vi "save_spectroscopy_hdf.vi"(3 "System Information cluster":T1, 5 "Subject metadata cluster":T2, 7 "Device Name":tag="DAQ2", 8 "Spectroscopy cluster in":T4, 9 "TxRxParams":T3={"sample rate"=1000000.0, "Transmit frequency"=25000.0, "Transmit amplitude"=1.577, "sample rate digital out"=40000.0, "TX cycles"=600, "sample rate DAQ1"=1000000.0, "Receive frequency"=75000.0, "Receive range"=1.0, "TX harmonics"=[50000.0, 75000.0, 100000.0, 125000.0, 150000.0, 175000.0, 200000.0, 225000.0]} {"TX harmonics" format="%#_6p"; "Receive frequency" format="%#_6p"; "sample rate DAQ1" format="%#_6p"; "sample rate digital out" format="%#_6p"; "Transmit frequency" format="%#_6p"; "sample rate" format="%#_6p"}, 11 "file path":path) -> ()   [LabVIEW 2021]
uses:
  <vilib>/UPVI/lvhdf5/file.llb/LVH5F Operation.ctl
  <vilib>/Utility/miscctls.llb/LVRectTypeDef.ctl
  <vilib>/UPVI/lvhdf5/group.llb/H5G_obj_t.ctl
  <vilib>/UPVI/lvhdf5/dataset.llb/LVH5D Operation.ctl
  <vilib>/UPVI/lvhdf5/attribute.llb/LVH5A Operation.ctl
  <vilib>/UPVI/lvhdf5/identifier.llb/Not an HDF5 Refnum Constant.vi
  <vilib>/UPVI/lvhdf5/attribute.llb/Write Multiple Attributes.vi
  <vilib>/UPVI/lvhdf5/utility.llb/Select HDF5 Dialog.vi
  <vilib>/UPVI/lvhdf5/utility.llb/Select HDF5 Dialog (Object Only).vi
  <vilib>/UPVI/lvhdf5/dataset.llb/Simple H5Dwrite (Variant).vi
  <vilib>/UPVI/lvhdf5/common.llb/To HDF5 Ref.vi
  <vilib>/UPVI/lvhdf5/dataset.llb/H5Dclose.vi
  <vilib>/UPVI/lvhdf5/attribute.llb/Simple H5Awrite (Variant).vi
  <vilib>/UPVI/lvhdf5/attribute.llb/LVH5 Write Attributes.xnode
  <vilib>/UPVI/lvhdf5/library.llb/HDF5 Ref.ctl
  <vilib>/UPVI/lvhdf5/dataset.llb/Simple H5Dwrite.xnode
  <vilib>/UPVI/lvhdf5/dataset.llb/Write Dataset with Attributes.xnode
  <vilib>/UPVI/lvhdf5/attribute.llb/Simple H5Awrite.xnode
  <vilib>/UPVI/lvhdf5/attribute.llb/Cluster to Attribute Array.xnode
  <vilib>/Utility/error.llb/Error Cluster From Error Code.vi
  <vilib>/UPVI/lvhdf5/dataset.llb/OpenCreateReplace Dataset by Element Type.vi
  <vilib>/UPVI/lvhdf5/dataspace.llb/H5Sselect_hyperslab.vi
  <vilib>/UPVI/lvhdf5/dataset.llb/H5Dwrite (Variant).vi
  <vilib>/UPVI/lvhdf5/dataset.llb/H5Dget_space.vi
  <vilib>/UPVI/lvhdf5/attribute.llb/private/LVH5AwriteWDTAttrs.vi
  <vilib>/UPVI/lvhdf5/dataspace.llb/H5Sclose.vi
  <vilib>/UPVI/lvhdf5/utility.llb/Select HDF5 Dialog (File and Object).vi
  <resource>/objmgr/daqmx.rc
  <vilib>/UPVI/lvhdf5/library.llb/HDF5 Ref.lvclass
  <vilib>/Utility/Data Type/Get Type Information.vi
  <vilib>/Utility/Data Type/NI_Data Type.lvlib
  <vilib>/Utility/Data Type/Get Cluster Information.vi
panel:
  out "proj mag f2-f9":dbl[][](array[numeric])
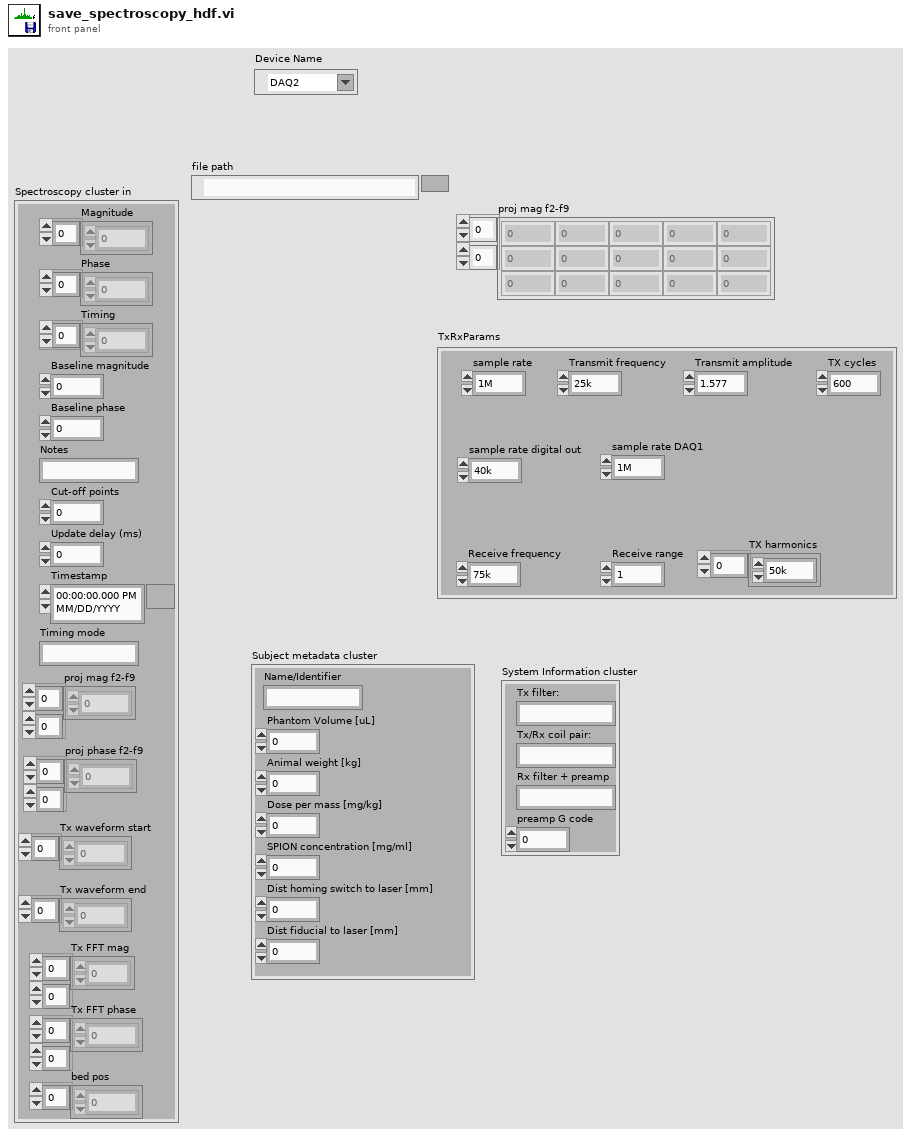
[diagram p1: front panel]
types:
  T1 = cluster{"Tx filter:":string, "Tx/Rx coil pair:":string, "Rx filter + preamp":string, "preamp G code":dbl}
  T2 = cluster{"Name/Identifier":string, "Phantom Volume [uL]":dbl, "Animal weight [kg]":dbl, "Dose per mass [mg/kg]":dbl, "SPION concentration [mg/ml]":dbl, "Dist homing switch to laser [mm]":dbl, "Dist fiducial to laser [mm]":dbl}
  T3 = cluster{"sample rate":dbl, "Transmit frequency":dbl, "Transmit amplitude":dbl, "sample rate digital out":dbl, "TX cycles":i32, "sample rate DAQ1":dbl, "Receive frequency":dbl, "Receive range":dbl, "TX harmonics":dbl[]}
  T4 = cluster{"Magnitude":dbl[], "Phase":dbl[], "Timing":dbl[], "Baseline magnitude":dbl, "Baseline phase":dbl, "Notes":string, "Cut-off points":i32, "Update delay (ms)":dbl, "Timestamp":timestamp, "Timing mode":string, "proj mag f2-f9":dbl[][], "proj phase f2-f9":dbl[][], "Tx waveform start":dbl[], "Tx waveform end":dbl[], "Tx FFT mag":dbl[][], "Tx FFT phase":dbl[][], "bed pos":dbl[]}
  T5 = typedef "LVH5F Operation.ctl" = enum16{"open", "open or create", "create or replace", "create or replace (with confirmation)", "create", "open (read only)"}
  T6 = typedef "HDF5 Ref.ctl" = refnum<class "HDF5 Ref.lvclass">
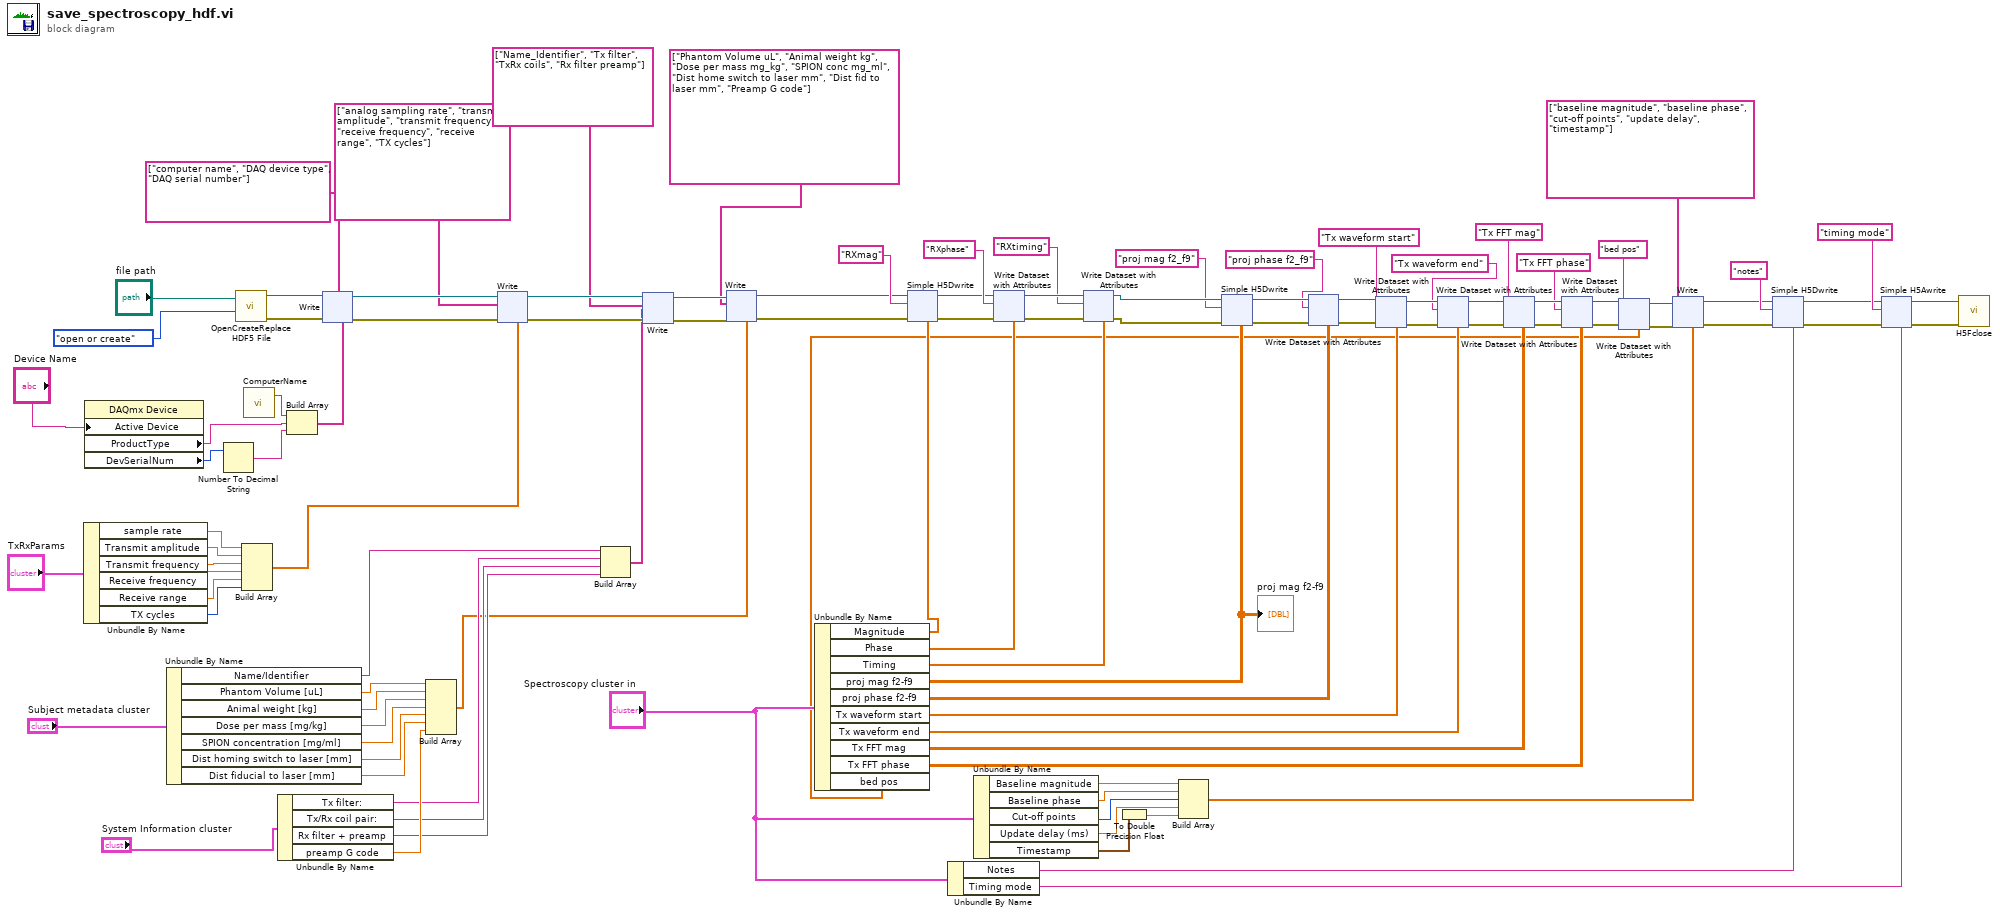
[diagram p0: block diagram]
diagram:
  n1 = Unbundle By Name("TxRxParams") -> ("sample rate"=w24:dbl, "Transmit amplitude"=w25:dbl, "Transmit frequency"=w26:dbl, "Receive frequency"=w27:dbl, "Receive range"=w28:dbl, "TX cycles"=w29:i32)
  n2 = property class="DAQmx Device"("Active Device"="Device Name") -> ("ProductType"=w95:string, "DevSerialNum"=w97:u32)  [unwired: 2 in, 2 out]
  n3 = Unbundle By Name("Subject metadata cluster") -> ("Name/Identifier"=w11:string, "Phantom Volume [uL]"=w17:dbl, "Animal weight [kg]"=w16:dbl, "Dose per mass [mg/kg]"=w15:dbl, "SPION concentration [mg/ml]"=w14:dbl, "Dist homing switch to laser [mm]"=w13:dbl, "Dist fiducial to laser [mm]"=w12:dbl)
  n4 = Number To Decimal String(number=w97) -> (decimal integer string=w96:string)  [unwired: 1 in]
  n5 = call <vilib>:"OpenCreateReplace HDF5 File.vi"("function (open or create)"=LVH5F_Operation."open or create", "path"="file path") -> ("error out"=w86:errorcluster, "HDF5 Ref out"=w87:T6)  [unwired: 6 in]
  n6 = Build Array(w24, w25, w26, w27, w28, w29) -> (w91:dbl[])
  n7 = call "ComputerName.vi"() -> ("String/Binary data"=w94:string)  [unwired: 4 in, 1 out]
  n8 = Unbundle By Name("System Information cluster") -> ("Tx filter:"=w9:string, "Tx/Rx coil pair:"=w8:string, "Rx filter + preamp"=w7:string, "preamp G code"=w10:dbl)
  n9 = Build Array(w94, w95, w96) -> (w93:string[])
  n10 = xnode "Write"("HDF5 Ref"=w87, "error in (no error)"=w86, "Name(s)"=string[] ["computer name", "DAQ device type", "DAQ serial number"], "Value(s)"=w93) -> ("HDF5 Ref out"=w85:T6, "error out"=w84:errorcluster)  [unwired: 1 in]
  n11 = Build Array(w17, w16, w15, w14, w13, w12, w10) -> (w3:dbl[])
  n12 = xnode "Write"("HDF5 Ref"=w85, "error in (no error)"=w84, "Name(s)"=string[] ["analog sampling rate", "transmit amplitude", "transmit frequency", "receive frequency", "receive range", "TX cycles"], "Value(s)"=w91) -> ("HDF5 Ref out"=w23:T6, "error out"=w21:errorcluster)  [unwired: 1 in]
  n13 = Build Array(w11, w9, w8, w7) -> (w4:string[])
  n14 = xnode "Write"("HDF5 Ref"=w23, "error in (no error)"=w21, "Name(s)"=string[] ["Name_Identifier", "Tx filter", "TxRx coils", "Rx filter preamp"], "Value(s)"=w4) -> ("HDF5 Ref out"=w22:T6, "error out"=w20:errorcluster)  [unwired: 1 in]
  n15 = xnode "Write"("HDF5 Ref"=w22, "error in (no error)"=w20, "Name(s)"=string[] ["Phantom Volume uL", "Animal weight kg", "Dose per mass mg_kg", "SPION conc mg_ml", "Dist home switch to laser mm", "Dist fid to laser mm", "Preamp G code"], "Value(s)"=w3) -> ("HDF5 Ref out"=w18:T6, "error out"=w19:errorcluster)  [unwired: 1 in]
  n16 = Unbundle By Name("Spectroscopy cluster in") -> ("Magnitude"=w82:dbl[], "Phase"=w81:dbl[], "Timing"=w78:dbl[], "proj mag f2-f9"=w56:dbl[][], "proj phase f2-f9"=w53:dbl[][], "Tx waveform start"=w46:dbl[], "Tx waveform end"=w45:dbl[], "Tx FFT mag"=w38:dbl[][], "Tx FFT phase"=w37:dbl[][], "bed pos"=w31:dbl[])
  "proj mag f2-f9" <- w56
  n17 = xnode "Simple H5Dwrite"("Dataset Path"="RXmag", "error in (no error)"=w19, "HDF5 Path or Ref"=w18, "Data"=w82) -> ("HDF5 Ref out"=w99:T6, "error out"=w100:errorcluster)  [unwired: 4 in, 1 out]
  n18 = Unbundle By Name("Spectroscopy cluster in") -> ("Notes"=w71:string, "Timing mode"=w65:string)
  n19 = Unbundle By Name("Spectroscopy cluster in") -> ("Baseline magnitude"=w76:dbl, "Baseline phase"=w75:dbl, "Cut-off points"=w74:i32, "Update delay (ms)"=w73:dbl, "Timestamp"=w64:timestamp)
  n20 = xnode "Write Dataset with Attributes"("Dataset Path"="RXphase", "error in (no error)"=w100, "HDF5 Path or Ref"=w99, "Data"=w81) -> ("HDF5 Ref out"=w80:T6, "error out"=w79:errorcluster)  [unwired: 4 in, 1 out]
  n21 = xnode "Write Dataset with Attributes"("Dataset Path"="RXtiming", "error in (no error)"=w79, "HDF5 Path or Ref"=w80, "Data"=w78) -> ("HDF5 Ref out"=w60:T6, "error out"=w58:errorcluster)  [unwired: 4 in, 1 out]
  n22 = To Double Precision Float(number=w64) -> (double precision float=w63:dbl)
  n23 = Build Array(w76, w75, w74, w73, w63) -> (w103:dbl[])
  n24 = xnode "Simple H5Dwrite"("Dataset Path"="proj mag f2_f9", "error in (no error)"=w58, "HDF5 Path or Ref"=w60, "Data"=w56) -> ("HDF5 Ref out"=w59:T6, "error out"=w57:errorcluster)  [unwired: 4 in, 1 out]
  n25 = xnode "Write Dataset with Attributes"("Dataset Path"="proj phase f2_f9", "error in (no error)"=w57, "HDF5 Path or Ref"=w59, "Data"=w53) -> ("HDF5 Ref out"=w52:T6, "error out"=w51:errorcluster)  [unwired: 4 in, 1 out]
  n26 = xnode "Write Dataset with Attributes"("Dataset Path"="Tx waveform start", "error in (no error)"=w51, "HDF5 Path or Ref"=w52, "Data"=w46) -> ("HDF5 Ref out"=w50:T6, "error out"=w49:errorcluster)  [unwired: 4 in, 1 out]
  n27 = xnode "Write Dataset with Attributes"("Dataset Path"="Tx waveform end", "error in (no error)"=w49, "HDF5 Path or Ref"=w50, "Data"=w45) -> ("HDF5 Ref out"=w42:T6, "error out"=w43:errorcluster)  [unwired: 4 in, 1 out]
  n28 = xnode "Write Dataset with Attributes"("Dataset Path"="Tx FFT mag", "error in (no error)"=w43, "HDF5 Path or Ref"=w42, "Data"=w38) -> ("HDF5 Ref out"=w41:T6, "error out"=w44:errorcluster)  [unwired: 4 in, 1 out]
  n29 = xnode "Write Dataset with Attributes"("Dataset Path"="Tx FFT phase", "error in (no error)"=w44, "HDF5 Path or Ref"=w41, "Data"=w37) -> ("HDF5 Ref out"=w34:T6, "error out"=w33:errorcluster)  [unwired: 4 in, 1 out]
  n30 = xnode "Write Dataset with Attributes"("Dataset Path"="bed pos", "error in (no error)"=w33, "HDF5 Path or Ref"=w34, "Data"=w31) -> ("HDF5 Ref out"=w36:T6, "error out"=w35:errorcluster)  [unwired: 4 in, 1 out]
  n31 = xnode "Write"("HDF5 Ref"=w36, "error in (no error)"=w35, "Name(s)"=string[] ["baseline magnitude", "baseline phase", "cut-off points", "update delay", "timestamp"], "Value(s)"=w103) -> ("HDF5 Ref out"=w70:T6, "error out"=w69:errorcluster)  [unwired: 1 in]
  n32 = xnode "Simple H5Dwrite"("Dataset Path"="notes", "error in (no error)"=w69, "HDF5 Path or Ref"=w70, "Data"=w71) -> ("HDF5 Ref out"=w67:T6, "error out"=w66:errorcluster)  [unwired: 4 in, 1 out]
  n33 = xnode "Simple H5Awrite"("HDF5 Ref"=w67, "Name"="timing mode", "error in (no error)"=w66, "Value"=w65) -> ("HDF5 Ref out"=w62:T6, "error out"=w61:errorcluster)  [unwired: 1 in]
  n34 = call <vilib>:"H5Fclose.vi"("error in (no error)"=w61, "HDF5 Ref"=w62) -> ()  [unwired: 7 in, 1 out]
